vi "Th_stopwatch.vi"() -> ()   [LabVIEW 2018]
uses:
  Th_GUI.vi
panel:
  out "数値 2":dbl format="%<%H:%M:%S%3u>t"
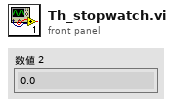
[diagram p1: front panel]
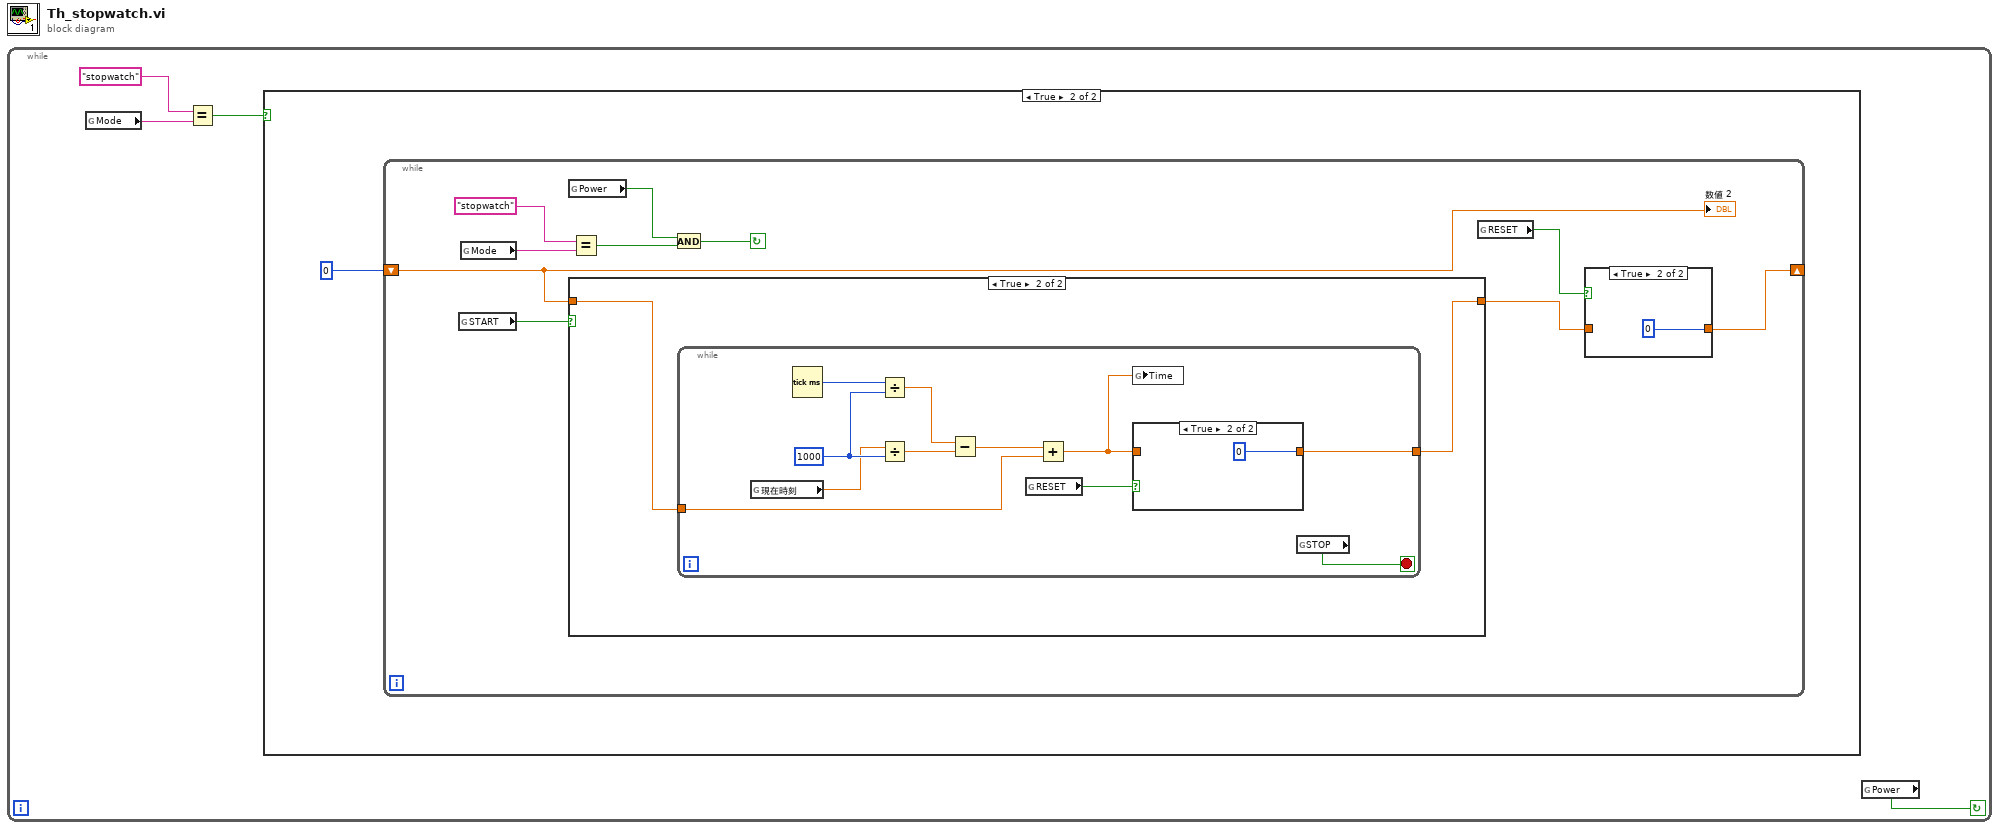
[diagram p0: block diagram]
diagram:
  n1 = while {
    stop <- w1 continue-if-true
    n2 = global read "Th_GUI.vi" "Mode"() -> (w4:string)
    n3 = Equal?(x="stopwatch", y=w4) -> (x = y?=w2:bool)
    n4 = case shown="TRUE" w2 {
      frame False {
      }
      frame True {
        n5 = while {
          shift-right: [w12] -> _
          shift-left: 0 -> [w15]
          stop <- w8 continue-if-true
          n6 = global read "Th_GUI.vi" "START"() -> (w14:bool)
          n7 = global read "Th_GUI.vi" "Mode"() -> (w10:string)
          n8 = global read "Th_GUI.vi" "Power"() -> (w7:bool)
          n9 = case shown="TRUE" w14 {
            tunnel: [w18 w19] -> w11
            tunnel: w15 -> [w18 w20]
            frame False {
            }
            frame True {
              n10 = while {
                tunnel: w20 -> [w26]
                tunnel: [w23] -> w19
                stop <- w25 stop-if-true
                w31 = 1000
                n11 = global read "Th_GUI.vi" "現在時刻"() -> (w24:dbl)
                n12 = Tick Count (ms)() -> (millisecond timer value=w30:u32)
                n13 = Divide(x=w30, y=w31) -> (x/y=w29:dbl)
                n14 = Divide(x=w24, y=w31) -> (x/y=w28:dbl)
                n15 = Subtract(x=w29, y=w28) -> (x-y=w27:dbl)
                n16 = global read "Th_GUI.vi" "RESET"() -> (w21:bool)
                n17 = Add(x=w27, y=w26) -> (x+y=w22:dbl)
                n18 = global write "Th_GUI.vi" "Time"(w22) -> ()
                n19 = case shown="TRUE" w21 {
                  tunnel: [w32 0] -> w23
                  tunnel: w22 -> [w32 _]
                  frame False {
                  }
                  frame True {
                  }
                }
                n20 = global read "Th_GUI.vi" "STOP"() -> (w25:bool)
              }
            }
          }
          n21 = Equal?(x="stopwatch", y=w10) -> (x = y?=w6:bool)
          n22 = And(x=w7, y=w6) -> (x .and. y?=w8:bool)
          n23 = global read "Th_GUI.vi" "RESET"() -> (w13:bool)
          n24 = case shown="TRUE" w13 {
            tunnel: [w16 0] -> w12
            tunnel: w11 -> [w16 _]
            frame False {
            }
            frame True {
            }
          }
          "数値 2" <- w15
        }
      }
    }
    n25 = global read "Th_GUI.vi" "Power"() -> (w1:bool)
  }
